vi "BT Example 2 - Sequence.vi"() -> ()   [LabVIEW 2021]
uses:
  Support/Nodes/abs_Node/Status.ctl
  Blackboard/Blackboard.lvclass
  Support/Nodes/Decorators/Repeater/Support/Finish On - Type.ctl
  System/bt_System.lvclass
  Blackboard/Blackboard.lvclass/Blackboard.ctl
  Blackboard/Get Value Type/Get Boolean.vi
  Blackboard/Support/Index Group.vi
  Blackboard/Support/Index Tags.vi
  <vilib>/TSA/Abstract Data Classes/Abs_Types/Boolean/Abs_Boolean.lvclass
  C:/Program Files (x86)/National Instruments/LabVIEW 2021/vi.lib/TSA/Abstract Data Classes/Abs_Types/Value/Abs_Value.lvclass
  <vilib>/TSA/Omni-Bus/Local Bus/Support/Bool/Local Bus_Boolean.lvclass
  <vilib>/TSA/Omni-Bus/Local Bus/Support/Initialise DVR's.vi
  <vilib>/TSA/Abstract Data Classes/Constants/Support/Bool/Bool.vi
  <vilib>/TSA/Abstract Data Classes/Abs_Types/Value/Abs_Value.lvclass
  <vilib>/TSA/Abstract Data Classes/Abs_Types/Type/Abs_Type.lvclass
  <vilib>/TSA/Omni-Bus/Local Bus/Support/DBL/Local Bus_DBL.lvclass
  <vilib>/TSA/Omni-Bus/Local Bus/Support/SGL/Local Bus_SGL.lvclass
  <vilib>/TSA/Omni-Bus/Local Bus/Support/EXT/Local Bus_EXT.lvclass
  <vilib>/TSA/Omni-Bus/Local Bus/Support/STR/Local Bus_String.lvclass
  <vilib>/TSA/Omni-Bus/Local Bus/Support/Variant/Local Bus_Variant.lvclass
  <vilib>/TSA/Omni-Bus/Local Bus/Support/WFM/Local Bus_Waveform.lvclass
  <vilib>/TSA/Omni-Bus/Local Bus/Support/Time/Local Bus_Time.lvclass
  <vilib>/TSA/Omni-Bus/Local Bus/Support/U8/Local Bus_U8.lvclass
  <vilib>/TSA/Omni-Bus/Local Bus/Support/U16/Local Bus_U16.lvclass
  <vilib>/TSA/Omni-Bus/Local Bus/Support/U32/Local Bus_U32.lvclass
  <vilib>/TSA/Omni-Bus/Local Bus/Support/U64/Local Bus_U64.lvclass
  <vilib>/TSA/Omni-Bus/Local Bus/Support/I8/Local Bus_I8.lvclass
  <vilib>/TSA/Omni-Bus/Local Bus/Support/I16/Local Bus_I16.lvclass
  <vilib>/TSA/Omni-Bus/Local Bus/Support/I32/Local Bus_I32.lvclass
  <vilib>/TSA/Omni-Bus/Local Bus/Support/I64/Local Bus_I64.lvclass
  <vilib>/TSA/Omni-Bus/Local Bus/Support/CSGL/Local Bus_CSGL.lvclass
  <vilib>/TSA/Omni-Bus/Local Bus/Support/CDBL/Local Bus_CDBL.lvclass
  <vilib>/TSA/Omni-Bus/Local Bus/Support/CEXT/Local Bus_CEXT.lvclass
  <vilib>/TSA/Abstract Data Classes/Abs_Types/Boolean/Static Read.vi
  BT.lvlib
  Support/Nodes/Decorators/Repeater/bt_Repeater.lvclass
  <vilib>/TSA/Abstract Data Classes/Constants/Support/Bool/Const_Bool.lvclass
  Support/Nodes/abs_Node/bt_Node.lvclass
panel:
  out "Status":T1
  out "Indicators":bool[](array[boolean])
  in  "stop":bool
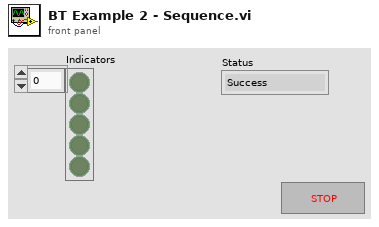
[diagram p1: front panel]
types:
  T1 = typedef "BT.lvlib/bt_Node.lvclass/Status.ctl" = enum16{"Success", "Failure", "Running"}
  T2 = typedef "BT.lvlib/bt_Repeater.lvclass/Finish On - Type.ctl" = enum16{"Success", "Failure", "Never"}
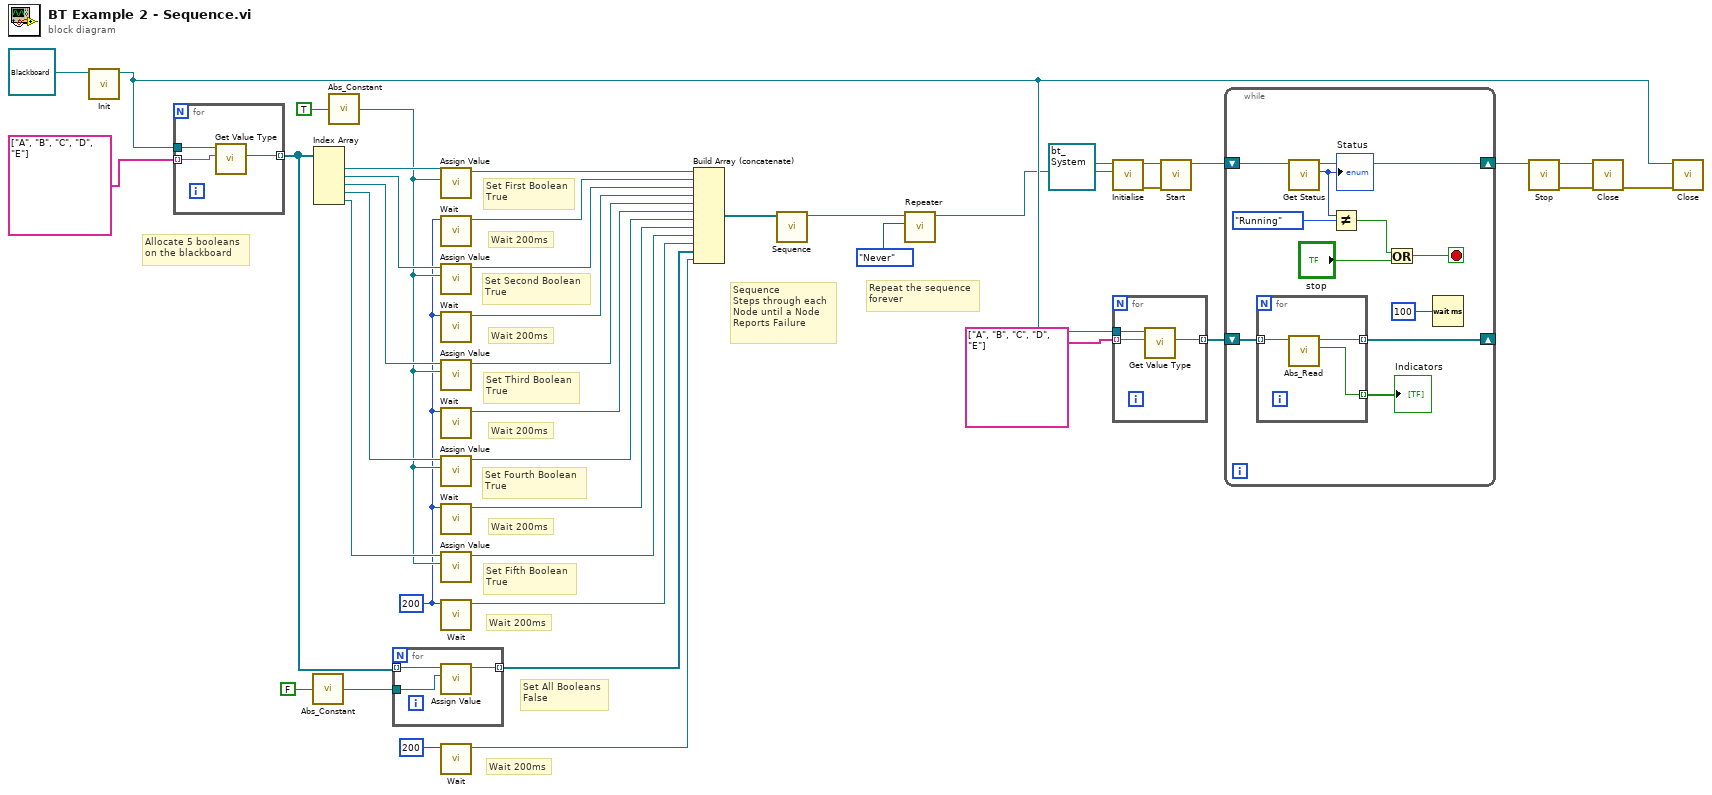
[diagram p0: block diagram]
diagram:
  w7 = u32 200 ("Time (ms)")
  # "Wait 200ms"
  # "Wait 200ms"
  # "Wait 200ms"
  # "Wait 200ms"
  # "Wait 200ms"
  # "Wait 200ms"
  # "Set All Booleans\nFalse"
  # "Set Fifth Boolean\nTrue"
  # "Set Fourth Boolean\nTrue"
  # "Set Third Boolean\nTrue"
  # "Set Second Boolean\nTrue"
  # "Set First Boolean\nTrue"
  # "Allocate 5 booleans\non the blackboard"
  # "Repeat the sequence\nforever"
  # "Sequence\nSteps through each\nNode until a Node\nReports Failure"
  n1 = call-dynamic "Init.vi"("bt_Blackboard in"=refnum<class "Blackboard.lvclass"> refnum) -> ("bt_Blackboard out"=w34:refnum<class "Blackboard.lvclass">)  [unwired: 9 in, 1 out]
  n2 = for {
    tunnel: w34 -> [w44]
    tunnel: string[] ["A", "B", "C", "D", "E"] ("Tag") -> [w43] mode=indexing
    tunnel: [w42] -> w4 mode=indexing
    n3 = call-poly "Get Value Type.vi"("Tag"=w43, "Blackboard in"=w44) -> ("Value"=w42:refnum<class "Abs_Boolean.lvclass">)  [unwired: 6 in, 3 out]
  }
  n4 = call-poly <vilib>:"Abs_Constant.vi"("Boolean"=FALSE) -> ("Abs_Boolean.lvclass"=w6:refnum<class "Abs_Boolean.lvclass">)  [unwired: 4 in]
  n5 = Index Array(array=w4) -> (element #1=w23:refnum<class "Abs_Boolean.lvclass">, element #2=w20:refnum<class "Abs_Boolean.lvclass">, element #3=w17:refnum<class "Abs_Boolean.lvclass">, element #4=w15:refnum<class "Abs_Boolean.lvclass">, element #5=w14:refnum<class "Abs_Boolean.lvclass">)  [unwired: 5 in]
  n6 = call-poly <vilib>:"Abs_Constant.vi"("Boolean"=TRUE) -> ("Abs_Boolean.lvclass"=w13:refnum<class "Abs_Boolean.lvclass">)  [unwired: 4 in]
  n7 = for {
    tunnel: w6 -> [w47]
    tunnel: w4 -> [w46] mode=indexing
    tunnel: [w45] -> w3 mode=indexing
    n8 = call "Assign Value.vi"("Assigned Value"=w47, "Value"=w46) -> ("Node Out"=w45:refnum<class "bt_Node.lvclass">)  [unwired: 9 in]
  }
  n9 = call "Assign Value.vi"("Assigned Value"=w13, "Value"=w23) -> ("Node Out"=w24:refnum<class "bt_Node.lvclass">)  [unwired: 9 in]
  n10 = call "Wait.vi"("Time (ms)"=w7) -> ("Node Out"=w21:refnum<class "bt_Node.lvclass">)  [unwired: 10 in]
  n11 = call "Assign Value.vi"("Assigned Value"=w13, "Value"=w20) -> ("Node Out"=w19:refnum<class "bt_Node.lvclass">)  [unwired: 9 in]
  n12 = call "Wait.vi"("Time (ms)"=w7) -> ("Node Out"=w18:refnum<class "bt_Node.lvclass">)  [unwired: 10 in]
  n13 = call "Assign Value.vi"("Assigned Value"=w13, "Value"=w17) -> ("Node Out"=w16:refnum<class "bt_Node.lvclass">)  [unwired: 9 in]
  n14 = call "Wait.vi"("Time (ms)"=w7) -> ("Node Out"=w12:refnum<class "bt_Node.lvclass">)  [unwired: 10 in]
  n15 = call "Assign Value.vi"("Assigned Value"=w13, "Value"=w15) -> ("Node Out"=w11:refnum<class "bt_Node.lvclass">)  [unwired: 9 in]
  n16 = call "Wait.vi"("Time (ms)"=w7) -> ("Node Out"=w10:refnum<class "bt_Node.lvclass">)  [unwired: 10 in]
  n17 = call "Assign Value.vi"("Assigned Value"=w13, "Value"=w14) -> ("Node Out"=w9:refnum<class "bt_Node.lvclass">)  [unwired: 9 in]
  n18 = call "Wait.vi"("Time (ms)"=w7) -> ("Node Out"=w8:refnum<class "bt_Node.lvclass">)  [unwired: 10 in]
  n19 = call "Wait.vi"("Time (ms)"=u32 200) -> ("Node Out"=w2:refnum<class "bt_Node.lvclass">)  [unwired: 10 in]
  n20 = Build Array (concatenate)(w24, w21, w19, w18, w16, w12, w11, w10, w9, w8, w3, w2) -> (w26:refnum<class "bt_Node.lvclass">[])
  n21 = call "Sequence.vi"("Nodes"=w26) -> ("Node"=w27:refnum<class "bt_Node.lvclass">)  [unwired: 10 in]
  n22 = call "Repeater.vi"("Finish On"=Finish_On_-_Type."Never", "Node In"=w27) -> ("Node Out"=w29:refnum<class "bt_Node.lvclass">)  [unwired: 9 in]
  n23 = call "Initialise.vi"("Behaviour Tree"=w29, "bt_System in"=refnum<class "bt_System.lvclass"> refnum) -> ("error out"=w30:errorcluster, "bt_System out"=w31:refnum<class "bt_System.lvclass">)  [unwired: 8 in]
  n24 = for {
    tunnel: string[] ["A", "B", "C", "D", "E"] ("Tag") -> [w50] mode=indexing
    tunnel: [w49] -> w36 mode=indexing
    tunnel: w34 -> [w48]
    n25 = call-poly "Get Value Type.vi"("Tag"=w50, "Blackboard in"=w48) -> ("Value"=w49:refnum<class "Abs_Boolean.lvclass">)  [unwired: 6 in, 3 out]
  }
  n26 = call "Start.vi"("error in (no error)"=w30, "bt_System in"=w31) -> ("bt_System out"=w41:refnum<class "bt_System.lvclass">)  [unwired: 8 in, 1 out]
  n27 = while {
    shift-right: [w56] -> w40
    shift-left: w41 -> [w57]
    shift-right: [w60] -> _
    shift-left: w36 -> [w61]
    stop <- w54 stop-if-true
    n28 = for {
      tunnel: w61 -> [w64] mode=indexing
      tunnel: [w63] -> w60 mode=indexing
      tunnel: [w62] -> w59 mode=indexing
      n29 = call-poly <vilib>:"Abs_Read.vi"("Abs_Boolean in"=w64) -> ("Boolean"=w62:bool, "Abs_Boolean out"=w63:refnum<class "Abs_Boolean.lvclass">)  [unwired: 8 in, 1 out]
    }
    "Indicators" <- w59
    n30 = call "Get Status.vi"("bt_System in"=w57) -> ("Status"=w53:T1, "bt_System out"=w56:refnum<class "bt_System.lvclass">)  [unwired: 8 in, 1 out]
    "Status" <- w53
    n31 = Not Equal?(x=w53, y=Status."Running") -> (x != y?=w51:bool)
    n32 = Or(x=w51, y="stop") -> (x .or. y?=w54:bool)
    n33 = Wait (ms)(milliseconds to wait=u32 100) -> ()  [unwired: 1 out]
  }
  n34 = call "Stop.vi"("bt_System in"=w40) -> ("error out"=w32:errorcluster, "bt_System out"=w33:refnum<class "bt_System.lvclass">)  [unwired: 9 in]
  n35 = call-dynamic "Close.vi"("error in (no error)"=w32, "bt_System in"=w33) -> ("error out"=w39:errorcluster)  [unwired: 8 in, 1 out]
  n36 = call-dynamic "Close.vi"("error in (no error)"=w39, "bt_Blackboard in"=w34) -> ()  [unwired: 8 in, 2 out]
